vi "Open FrontPanel.vi"(0 "Task Setting Editor in":refnum<class "Task Setting Editor.lvclass">, 1 "Open":bool, 3 "error in (no error)":errorcluster) -> (7 "Task Setting Editor out":refnum<class "Task Setting Editor.lvclass">, 10 "error out":errorcluster)   [LabVIEW 2017, in "Task Setting Editor.lvlib" / "Task Setting Editor.lvclass"]
uses:
  Task Setting Editor.lvclass
  Task Setting Editor.lvclass/Task Setting Editor.ctl
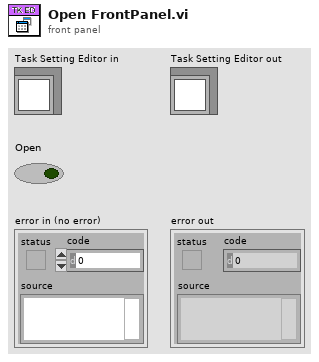
[diagram p1: front panel]
types:
  T1 = enum32{"Invalid", "Standard", "Closed", "Hidden", "Minimized", "Maximized"}
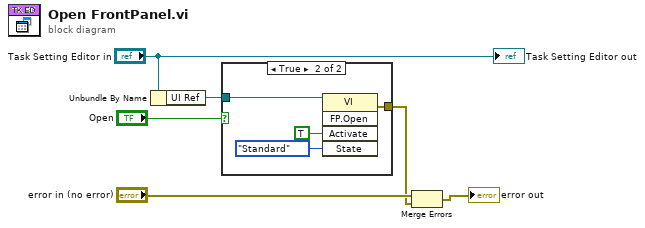
[diagram p0: block diagram]
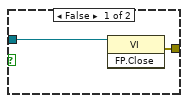
[diagram p2: hidden frame]
diagram:
  n1 = Unbundle By Name("Task Setting Editor in") -> ("UI Ref"=w1:refnum<vi>)
  n2 = case shown="True" "Open" {
    tunnel: w1 -> [w8 w10]
    tunnel: [w7 w9] -> w3
    frame False {
      n3 = invoke class="VI" method="FP.Close"(reference=w8) -> (error out=w7:errorcluster)  [unwired: 2 in, 2 out]
    }
    frame True {
      n4 = invoke class="VI" method="FP.Open"(reference=w10, "Activate"=TRUE ("Activate?"), "State"=T1."Standard") -> (error out=w9:errorcluster)  [unwired: 2 in, 4 out]
    }
  }
  n5 = Merge Errors("error in (no error)", w3) -> (→"error out":errorcluster)
  "Task Setting Editor out" <- "Task Setting Editor in"
